vi "Insert Column into Table.vi"(3 "Index":i32, 4 "Column in":dbl[](array[numeric]), 5 "Table in":dbl[][](array[numeric])) -> (2 "Table out":dbl[][](array[numeric]))   [LabVIEW 2018, in "Potentiostat Galvanostat.lvclass"]
uses:
  Potentiostat Galvanostat.lvclass
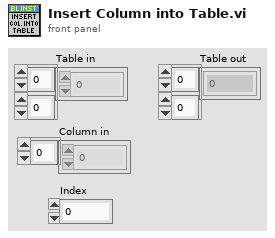
[diagram p1: front panel]
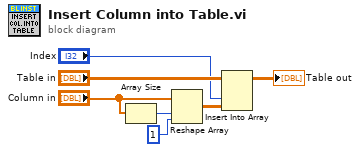
[diagram p0: block diagram]
diagram:
  n1 = Array Size(array="Column in") -> (size(s)=w5:i32)
  n2 = Reshape Array("Column in", w5, 1 ("dimension size")) -> (w3:dbl[][])
  n3 = Insert Into Array(array="Table in", index (col)="Index", new element=w3) -> (→"Table out":dbl[][])  [unwired: 1 in]
